vi "Dashboard Main - save.vi"() -> ()   [LabVIEW 2014]
uses:
  <vilib>/event_ctls.llb/eventvkey.ctl
  <vilib>/Utility/config.llb/NI_LVConfig.lvlib
  <vilib>/Utility/config.llb/Write Key (I32).vi
  <vilib>/Rock Robotics/WPI/Dashboard/WPI_DashboardLogging Global.vi
  <vilib>/Utility/config.llb/Write Key (String).vi
panel:
  in  "TCP":refnum<k5>
  in  "Rec Mode":enum32{"Stop", "Record", "Playback"}(radio)
  in  "Vision":u16(ring) items=["Camera Off", "USB Camera SW", "USB Camera HW", "IP Camera"]
  out "Camera IP":string
  out "Image Message":string="Timeout in Camera Communications"
  in  "Dashboard Tab":T1(tab)
  in  "Boolean":bool
  out "Low Battery":bool
  out "FMS":bool
  out "Teleop Mode":bool
  out "Auto Mode":bool
  out "Disabled":bool
  in  "Program":string
  in  "Camera Settings":T2={"Frame Rate"=30, "Compression"=30, "Size"=1} {"Frame Rate" scale=1.0..30.0; "Size" items=["640x480", "320x240", "160x120"]}
  out "Mode":T3(ring)=enum."Auto Disabled"
  in  "DB Camera Config":bool
  out "fps":dbl format="%#.1g"
  out "Mbps":dbl format="%#.1g"
  out "Mbps 2":bool
  in  "LCD Line 10":string caption="DB/String 0"
  in  "LCD Line 9":string caption="DB/String 0"
  in  "LCD Line 8":string caption="DB/String 0"
  in  "LCD Line 7":string caption="DB/String 0"
  in  "LCD Line 6":string caption="DB/String 0"
  in  "LCD Line 5":string caption="DB/String 0"
  in  "LCD Line 4":string caption="DB/String 0"
  in  "LCD Line 3":string caption="DB/String 0"
  in  "LCD Line 2":string caption="DB/String 0"
  in  "LCD Line 1":string caption="DB/String 0"
  in  "DB/String 9":string
  in  "DB/String 8":string
  in  "DB/String 7":string
  in  "DB/String 6":string
  in  "DB/String 5":string
  in  "DB/String 4":string
  in  "DB/String 3":string
  in  "DB/String 2":string
  in  "DB/String 1":string
  in  "DB/String 0":string
  in  "DB/Slider 0":dbl(slide) scale=0.0..5.0
  in  "DB/Slider 1":dbl(slide) scale=0.0..5.0
  in  "DB/Slider 2":dbl(slide) scale=0.0..5.0
  in  "DB/Slider 3":dbl(slide) scale=0.0..5.0
  out "DB/LED 3":bool
  out "DB/LED 2":bool
  out "DB/LED 1":bool
  out "DB/LED 0":bool
  in  "DB/Button 3":bool
  in  "DB/Button 2":bool
  in  "DB/Button 1":bool
  in  "DB/Button 0":bool caption="New Name"
  in  "Test Slider":dbl(slide) scale=0.0..100.0 scale format="%#_3g"
  in  "On/Off":bool caption="Solenoid"
  in  "Test Name":u16(ring) items=["Select the test to run...", "Example Test", "-------------------------------", "List of tests is built in robot code.", "Replace with your own automated tests."]
  in  "Test Tree":string(tree)
  in  "Motor":cluster{"Value":dbl, "Enable":bool} {"Value" scale=-1.0..1.0 scale format="%#_3g"}
  out "Progress":T4 {"Test Progress" scale=0.0..100.0}
  in  "Rev/Fwd":cluster{"Forward":bool, "Reverse":bool}
  in  "Test Ring":u16(ring) items=["Monochrome", "Color"]
  in  "Listbox":i32(listbox)
  out "Tree":string(tree)
  out "Camera Image":T5(plugin-control)
  # "Program:"
  # "Dashboard: 2015-02"
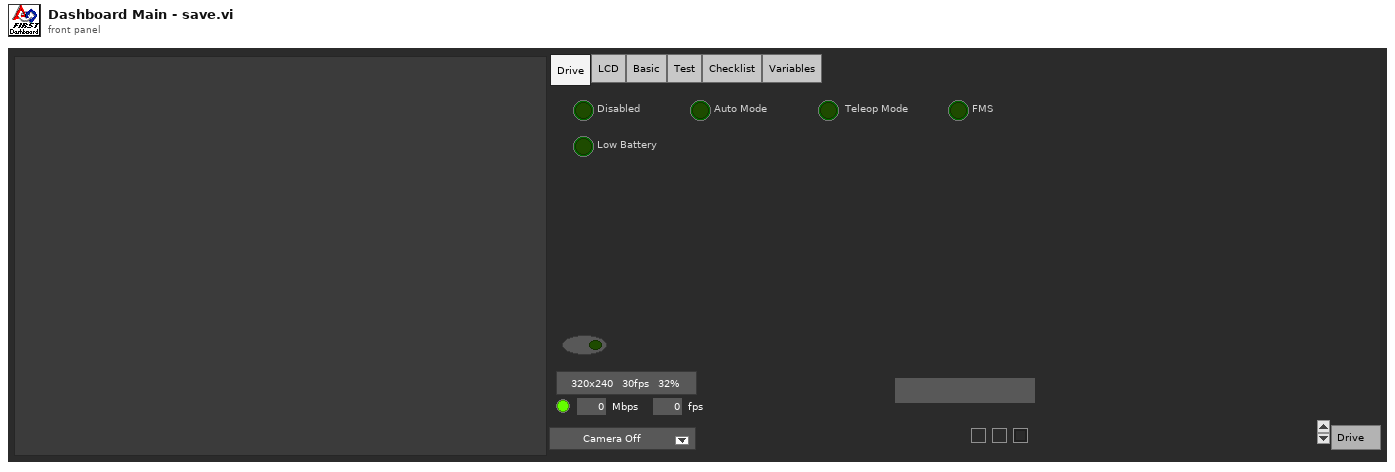
[diagram p1: front panel]
types:
  T1 = enum32{"Drive", "LCD", "Basic", "Test", "Checklist", "Variables"}
  T2 = cluster{"Frame Rate":i32, "Compression":i32, "Size":u16}
  T3 = enum8{"Tele-Op Disabled", "Tele-Op Enabled", "Auto Disabled", "Auto Enabled", "Test Disabled", "Test Enabled", "Disconnected", "No Code", "E-Stop"}
  T4 = cluster{"Test Progress":u8, "Test Progress Text":string}
  T5 = typedef "IMAQ Image.ctl" = refnum<image>
  T6 = enum32{"Drive", "Basic", "Custom", "Test", "Checklist", "Variables"}
  T7 = typedef "Image Type" = u32
  T8 = cluster{"Camera Image":refnum<vi>, "Dashboard Tab":refnum<vi>, "Vision":refnum<vi>, "Rec Mode":refnum<vi>, "Test Slider":refnum<vi>, "On/Off ":refnum<vi>, "Test Ring":refnum<vi>, "Rev/Fwd":refnum<vi>, "Test Name":refnum<vi>, "Motor":refnum<vi>, "Progress":refnum<vi>, "CheckList":refnum<vi>, "Tree":refnum<vi>, "Test Tree":refnum<vi>, void}
  T9 = cluster{"Error Strings":string, "Disable Counts":cluster{u16, u16}, "Rail Faults":cluster{u16, u16, u16}, "Robot IP":string, "DB Mode":u8, "Event Info":cluster{"Name":string, "Type":u8, "Number":u16, "Replay":u8}, "Camera Addr":string}
  T10 = cluster{"Storage":cluster{"Disk Free":u64, "RAM Block":u32, "RAM free":u32}, "CPU Utilization":cluster{"CPU % ISR":sgl, "CPU % Time Crit":sgl, "CPU % Timed Str":sgl, "CPU % High":sgl, "CPU % Above":sgl, "CPU % Normal":sgl, "CPU % Low":sgl}, "CAN":cluster{"% Bus Utilization":sgl, "Bus Off Cnt":u32, "TX_FIFO Full Cnt":u32, "Receive Error Cnt":u8, "Transmit Error Cnt":u8}, "HID":cluster{"HID Outputs":u32, "Rumble Low":u16, "Rumble High":u16}[]}
  T11 = cluster{"Status bits":cluster{"Test Mode":bool, "Autonomous":bool, "Enabled":bool, "Code Start":bool, "Brownout":bool, "Reserved 2":bool, "Reserved 3":bool, "E-Stop":bool}, "Code Trace":cluster{"Disabled":bool, "TeleOp":bool, "Auto":bool, "Test":bool}, "Controller Type":enum16{"unknown", "cRIO", "roboRio"}, "Code?":enum16{"unknown", "noCode", "code"}, "Battery V":dbl}
  T12 = cluster{"Control Bits":cluster{"TestMode":bool, "Autonomous":bool, "Enabled":bool, "FMS Present":bool, bool, bool, bool, "E-Stop":bool}, "Team Station ":u8, "Countdown":sgl, "Joystick Values":cluster{"Axes":dbl[], "Buttons":bool[], "POVs":i16[]}[]}
  T13 = cluster{"Axes":dbl[], "Buttons":bool[], "POVs":i16[]}[]
  T14 = cluster{"Axes":dbl[], "Buttons":bool[], "POVs":i16[]}
  T15 = typedef "NI_LVConfig.lvlib/Config Data RefNum.ctl" = refnum<k1>
  T16 = cluster{"Operation":enum16{"Update", "Clear"}, "Color Box":u32}[]
  T17 = typedef "eventvkey.ctl" = enum16{"ASCII", "Enter", "Return", "Shift", "Ctrl", "Alt", "Cmd", "Opt", "Caps", "NumLock", "Clear", "Break", "Up", "Down", "Left", "Right", "Insert", "Delete", "Home", "End", "PageUp", "PageDown", "Escape", "Help", "Pause", "ScrollLock", "F1", "F2", "F3", "F4", "F5", "F6", "F7", "F8", "F9", "F10", "F11", "F12", "F13", "F14", "F15", "F16", "F17", "F18", "F19", "F20", "F21", "F22", "F23", "F24", "Play", "VolumeUp", "VolumeDown", "Mute", "Two Byte Char"}
  T18 = cluster{"Image Size":bool, "Image Type":bool, "Pixel Value":bool, "ROI Information":bool, "Zoom Factor":bool}
  T19 = enum8{"Enabled", "Disabled", "Disabled and Grayed Out"}
  T20 = cluster{"Operation":enum16{"Update", "Clear"}, "Color Box":u32}
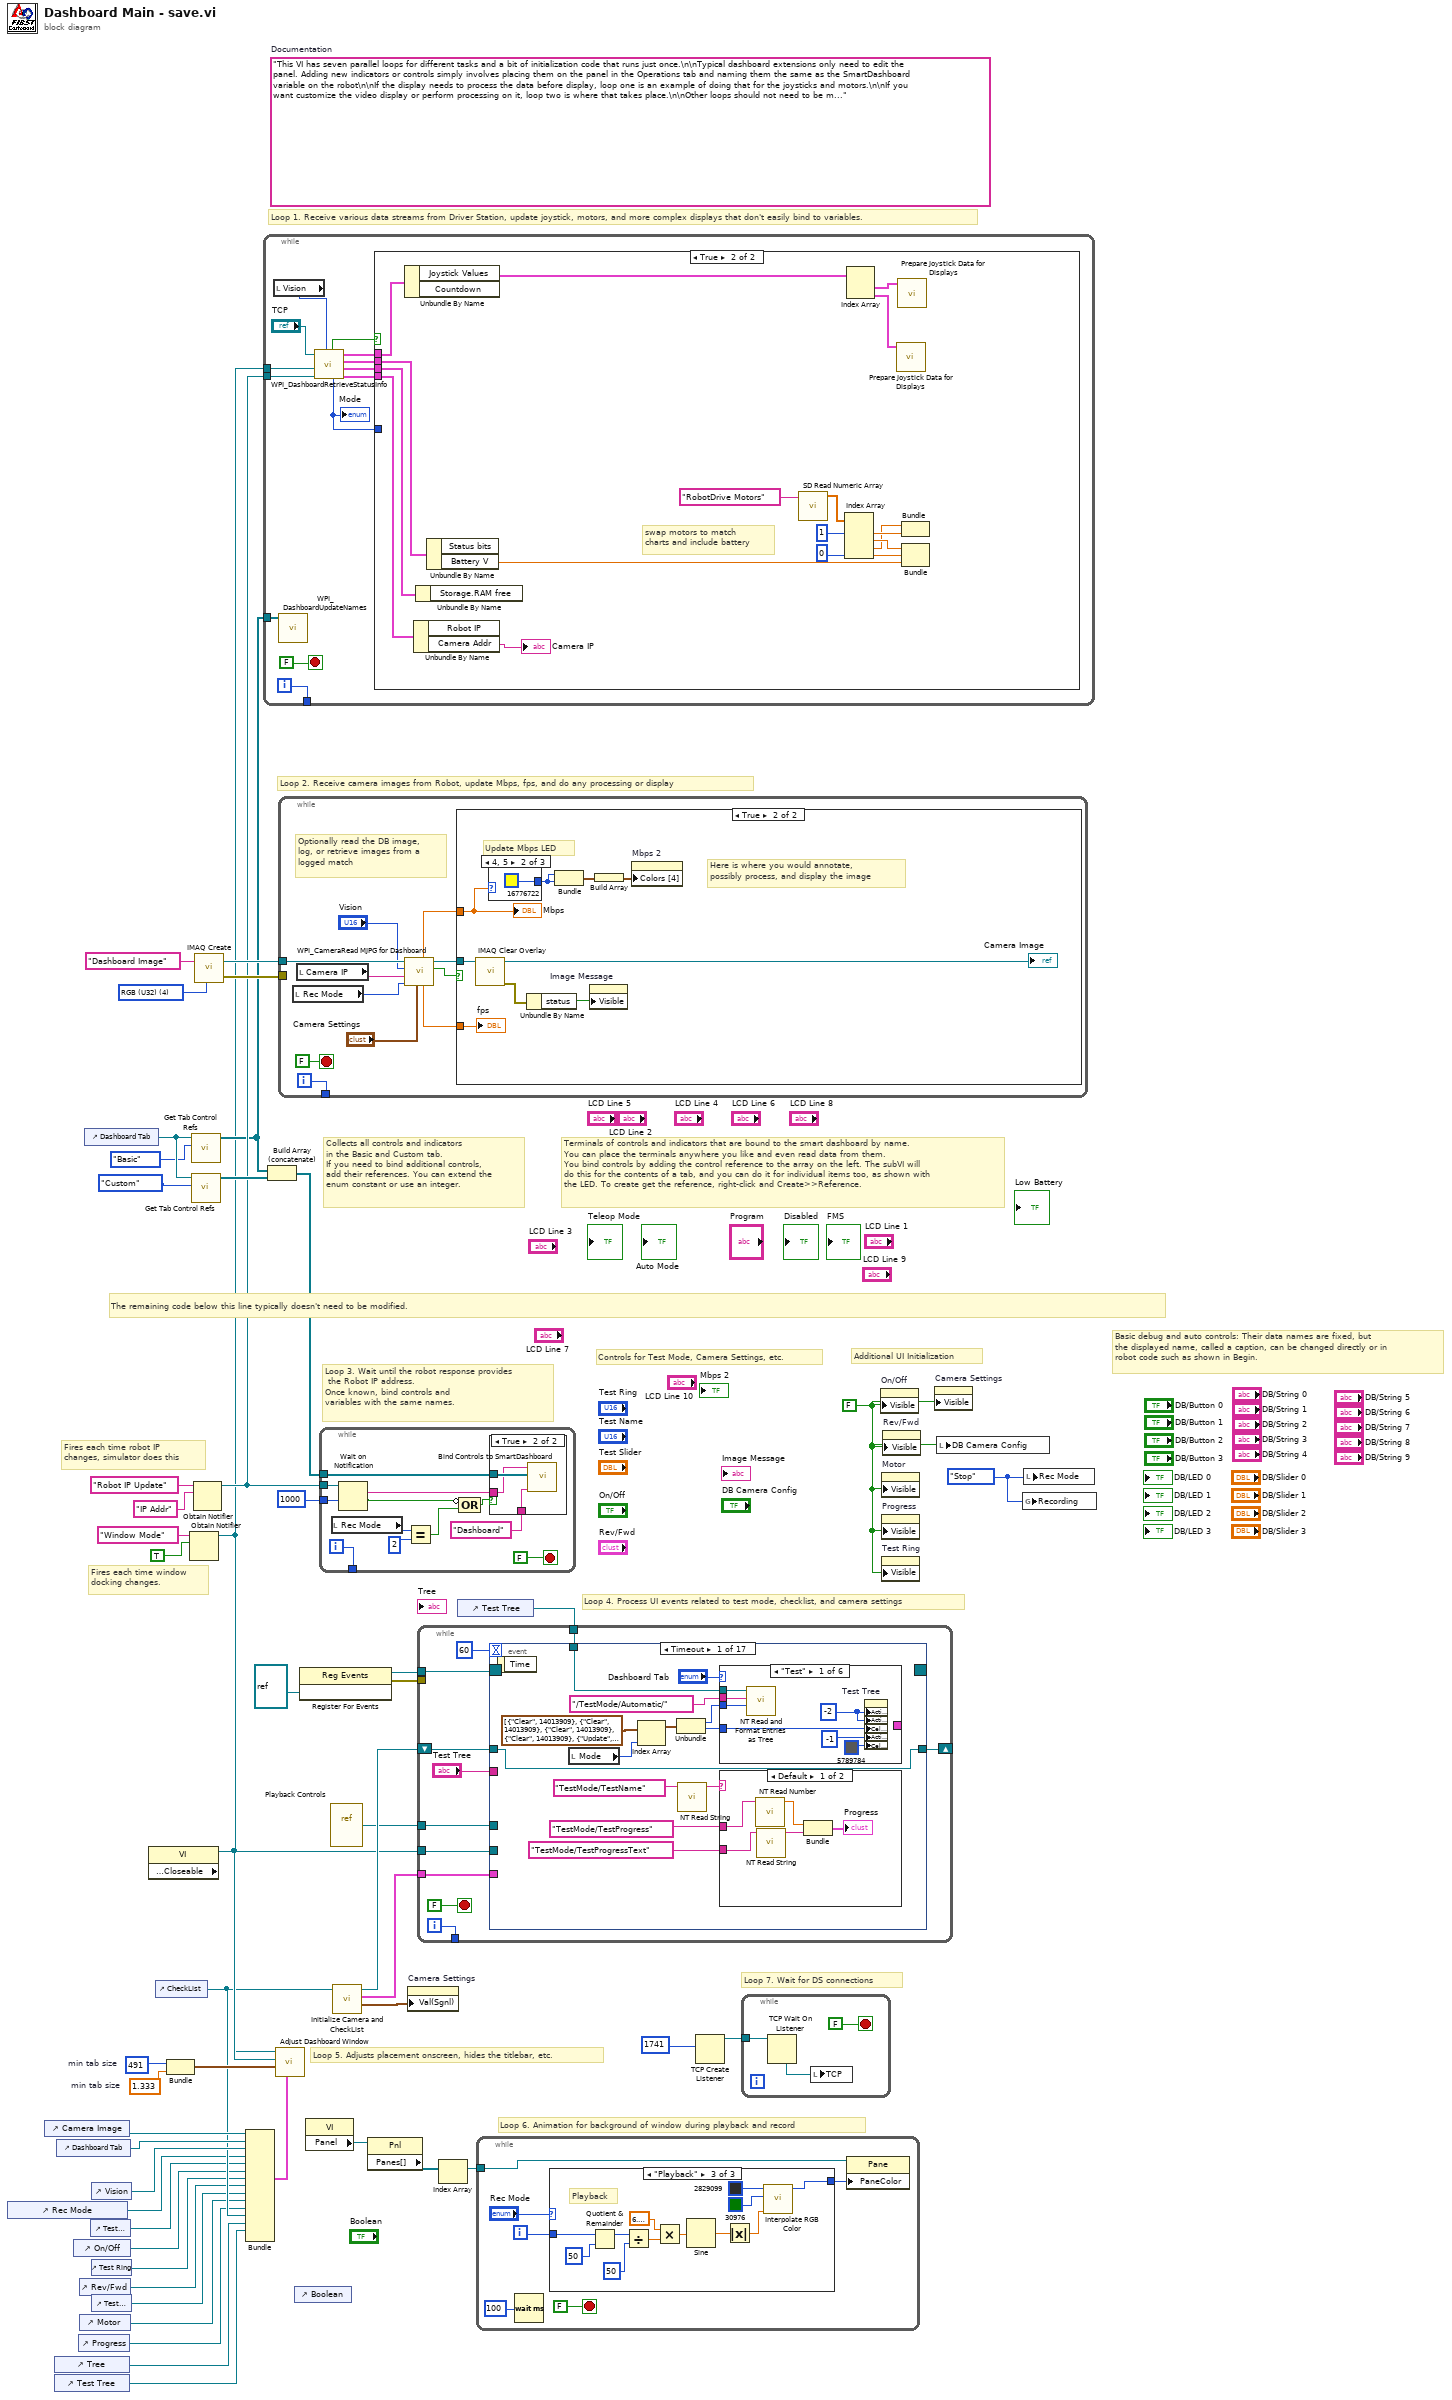
[diagram p0: block diagram]
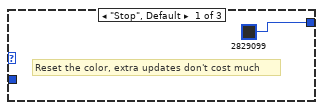
[diagram p3: hidden frame]
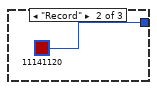
[diagram p4: hidden frame]
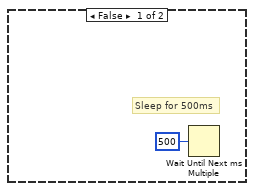
[diagram p6: hidden frame]
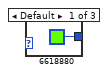
[diagram p7: hidden frame]
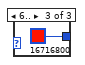
[diagram p8: hidden frame]
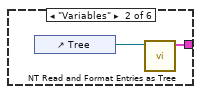
[diagram p9: hidden frame]
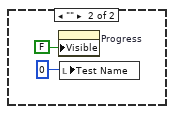
[diagram p14: hidden frame]
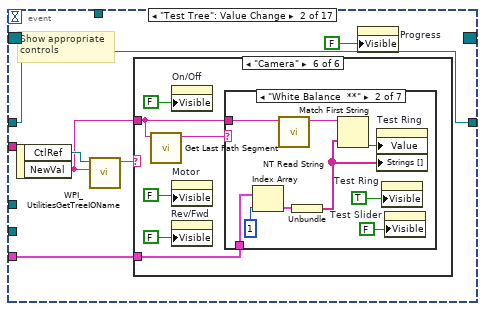
[diagram p15: hidden frame]
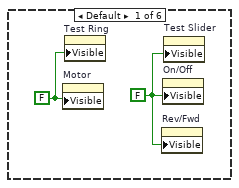
[diagram p16: hidden frame]
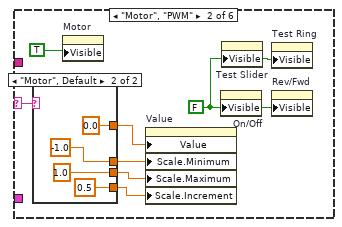
[diagram p17: hidden frame]
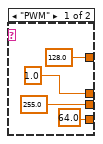
[diagram p18: hidden frame]
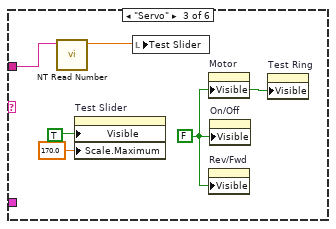
[diagram p19: hidden frame]
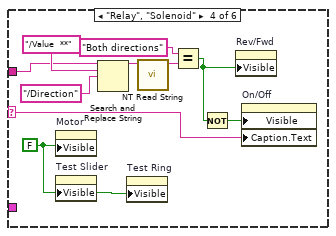
[diagram p20: hidden frame]
diagram:
  w23 = 491  # min tab size
  w22 = 1.333  # min tab size
  w31 = enum32{"Stop", "Record", "Playback"}."Stop" ("Rec Mode")
  w6 = FALSE ("Visible")
  (unwired) "This VI has seven parallel loops for different tasks and a bit of initialization code that runs just once.\n\nTypical dashboard extensions only need to edit the panel. Adding new indicators or controls simply involves placing them on the panel in the Operations tab and naming them the same as the SmartDashboard variable on the robot\n\nIf the display needs to process the data before display, loop one is an example of doing that for the joysticks and motors.\n\nIf you want customize the video display or perform processing on it, loop two is where that takes place.\n\nOther loops should not need to be modified. They are pretty standard, and document the task they perform."  # Documentation
  w51 = T7 4 items=["Grayscale (U8)", "Grayscale (I16)", "Grayscale (SGL)", "Complex (CSG)", "RGB (U32)", "HSL (U32)", "RGB (U64)"] ("Image Type")
  # "Loop 7. Wait for DS connections"
  # "Basic debug and auto controls: Their data names are fixed, but\nthe displayed name, called a caption, can be changed directly or in\nrobot code such as shown in Begin."
  # "Controls for Test Mode, Camera Settings, etc."
  # "Additional UI Initialization"
  # "Loop 6. Animation for background of window during playback and record"
  # "Fires each time robot IP\nchanges, simulator does this"
  # "Fires each time window\ndocking changes."
  # "Collects all controls and indicators\nin the Basic and Custom tab.\nIf you need to bind additional controls,\nadd their references. You can extend the\nenum constant or use an integer."
  # "The remaining code below this line typically doesn't need to be modified."
  # "Loop 4. Process UI events related to test mode, checklist, and camera settings"
  # "Terminals of controls and indicators that are bound to the smart dashboard by name.\nYou can place the terminals anywhere you like and even read data from them.\nYou bind controls by adding the control reference to the array on the left. The subVI will\ndo this for the contents of a tab, and you can do it for individual items too, as shown with\nthe LED. To create get the reference, right-click and Create>>Reference."
  # "Loop 3. Wait until the robot response provides\n the Robot IP address.\nOnce known, bind controls and\nvariables with the same names."
  # "Loop 5. Adjusts placement onscreen, hides the titlebar, etc."
  # "Loop 1. Receive various data streams from Driver Station, update joystick, motors, and more complex displays that don't easily bind to variables."
  # "Loop 2. Receive camera images from Robot, update Mbps, fps, and do any processing or display"
  n1 = control-ref of="Rec Mode"() -> (w12:refnum<vi>)
  n2 = control-ref of="Camera Image"() -> (w26:refnum<vi>)
  n3 = control-ref of="Tree"() -> (w16:refnum<vi>)
  n4 = control-ref of="Test Tree"() -> (w15:refnum<vi>)
  n5 = control-ref of="Dashboard Tab"() -> (w25:refnum<vi>)
  n6 = control-ref of="On/Off"() -> (w10:refnum<vi>)
  n7 = control-ref of="Progress"() -> (w7:refnum<vi>)
  n8 = control-ref of="Rev/Fwd"() -> (w8:refnum<vi>)
  n9 = control-ref of="Motor"() -> (w13:refnum<vi>)
  n10 = control-ref of="Dashboard Tab"() -> (w29:refnum<vi>)
  n11 = control-ref of="Test Slider"() -> (w11:refnum<vi>)
  n12 = control-ref of="Vision"() -> (w24:refnum<vi>)
  n13 = control-ref of="Test Ring"() -> (w9:refnum<vi>)
  n14 = control-ref of="Test Name"() -> (w14:refnum<vi>)
  n15 = property class="VI" props=["Front Panel.Closeable"]() -> (reference out=w30:refnum<vi>)  [unwired: 2 in, 2 out]
  n16 = control-ref of="CheckList"() -> (w17:refnum<vi>)
  n17 = Bundle("min tab size"=w23, "min tab size"=w22) -> (w21:cluster{"min tab size":i32, "min tab size":dbl})  [unwired: 1 in]
  n18 = Obtain Notifier(name (unnamed)="Window Mode", notification data type=TRUE) -> (notifier out=w3:refnum<notifier>)  [unwired: 2 in, 2 out]
  n19 = call <vilib>:"Get Tab Control Refs.vi"("Page Index"=T6."Basic" ("Dashboard Tab"), "TabControl in"=w29) -> ("ControlsOnPage"=w4:refnum<vi>[])  [unwired: 9 in]
  n20 = call <vilib>:"Get Tab Control Refs.vi"("Page Index"=T6."Custom" ("Dashboard Tab"), "TabControl in"=w29) -> ("ControlsOnPage"=w28:refnum<vi>[])  [unwired: 9 in]
  n21 = Obtain Notifier(name (unnamed)="Robot IP Update", notification data type="IP Addr" ("name (unnamed)")) -> (notifier out=w5:refnum<notifier>)  [unwired: 2 in, 2 out]
  n22 = call "IMAQ Create"("Image Name"="Dashboard Image", "Image Type"=w51) -> ("New Image"=w49:T5, "error out"=w48:errorcluster)  [unwired: 2 in, 1 out]
  n23 = Bundle("Camera Image"=w26, "Dashboard Tab"=w25, "Vision"=w24, "Rec Mode"=w12, "Test Slider"=w11, "On/Off"=w10, "Test Ring"=w9, "Rev/Fwd"=w8, "Test Name"=w14, "Motor"=w13, "Progress"=w7, "CheckList"=w17, "Tree"=w16, "Test Tree"=w15) -> (w18:T8)  [unwired: 2 in]
  n24 = while {
    tunnel: [w63] -> _
    tunnel: w5 -> [w57]
    tunnel: w4 -> [w56]
    tunnel: w3 -> [w52]
    i -> [w63]
    stop <- FALSE stop-if-true
    n25 = local read "Vision"() -> (w54:u16)
    n26 = call <vilib>:"WPI_DashboardUpdateNames.vi"("Controls on Tab"=w56) -> ()  [unwired: 11 in]
    n27 = call <vilib>:"WPI_DashboardRetrieveStatusInfo.vi"("Vision"=w54, "Binding Refnum"=w57, "Window Mode Notifier"=w52, "TCP Cnx"="TCP") -> ("Power and Errors"=w58:T9, "Robot Metrics"=w61:T10, "Status Info"=w62:T11, "Control Info"=w59:T12, "Robot Mode"=w55:T3, "Process?"=w60:bool)  [unwired: 2 in]
    "Mode" <- w55
    n28 = case shown="True" w60 {
      tunnel: w62 -> [_ w81]
      tunnel: w61 -> [_ w80]
      tunnel: w59 -> [_ w79]
      tunnel: w58 -> [_ w78]
      tunnel: w55 -> [_ _]
      frame False {
      }
      frame True {
        # "swap motors to match\ncharts and include battery"
        n29 = Unbundle By Name(w79) -> ("Joystick Values"=w68:T13)  [unwired: 1 out]
        n30 = Unbundle By Name(w78) -> ("Camera Addr"=→"Camera IP":string)  [unwired: 1 out]
        n31 = Unbundle By Name(w80) -> ()  [unwired: 1 out]
        n32 = Unbundle By Name(w81) -> ("Battery V"=w69:dbl)  [unwired: 1 out]
        n33 = call <vilib>:"SD Read Numeric Array.vi"("Name"="RobotDrive Motors") -> ("Numeric Array"=w71:dbl[])  [unwired: 8 in, 2 out]
        n34 = Index Array(array=w71, index #1=1, index #4=0) -> (element #1=w73:dbl, element #2=w74:dbl, element #3=w72:dbl, element #4=w77:dbl)  [unwired: 2 in]
        n35 = Index Array(array=w68) -> (element #1=w67:T14, element #2=w65:T14)  [unwired: 2 in]
        n36 = call "Prepare Joystick Data for Displays.vi"("Joystick Values"=w65) -> ()  [unwired: 8 in, 3 out]
        n37 = call "Prepare Joystick Data for Displays.vi"("Joystick Values"=w67) -> ()  [unwired: 8 in, 3 out]
        n38 = Bundle("Numeric"=w72, "Numeric"=w73) -> ()  [unwired: 1 in, 1 out]
        n39 = Bundle("Numeric"=w74, "Numeric"=w77, "Battery V"=w69) -> ()  [unwired: 1 in, 1 out]
      }
    }
  }
  n40 = Build Array (concatenate)(w4, w28) -> (w27:refnum<vi>[])
  n41 = call "Adjust Dashboard Window.vi"("Sizing Refnums"=w18, "Size Constraints"=w21, "VI"=w30, "Notifier in"=w3) -> ()  [unwired: 8 in]
  n42 = while {
    tunnel: w49 -> [w90]
    tunnel: w48 -> [_]
    tunnel: [w91] -> _
    i -> [w91]
    stop <- FALSE stop-if-true
    # "Optionally read the DB image,\nlog, or retrieve images from a\nlogged match"
    n43 = local read "Rec Mode"() -> (w84:enum32{"Stop", "Record", "Playback"})
    n44 = local read "Camera IP"() -> (w82:string)
    n45 = call <vilib>:"WPI_CameraRead MJPG for Dashboard.vi"("Camera Settings"="Camera Settings", "Rec Mode"=w84, "Camera IP"=w82, "Camera Mode"="Vision", "Refnum in"=w90) -> ("Active"=w88:bool, "Refnum out"=w89:T5, "FPS"=w87:dbl, "Bandwidth (Mbps)"=w86:dbl)  [unwired: 3 in]
    n46 = case shown="True" w88 {
      tunnel: w89 -> [_ w97]
      tunnel: w86 -> [_ w96]
      tunnel: w87 -> [_ w94]
      frame False {
        # "Sleep for 500ms"
        n47 = Wait Until Next ms Multiple(millisecond multiple=u32 500) -> ()  [unwired: 1 out]
      }
      frame True {
        # "Here is where you would annotate,\npossibly process, and display the image"
        # "Update Mbps LED"
        n48 = call "IMAQ Clear Overlay"("Image"=w97) -> ("error out"=w101:errorcluster, "Image Out"=→"Camera Image":T5)  [unwired: 2 in, 7 out]
        n49 = case shown="4, 5" w96 {
          tunnel: [u32 6618880 ("Color Box") u32 16776722 ("Color Box") u32 16716800 ("Color Box")] -> w98
          frame Default {
          }
          frame 4, 5 {
          }
          frame 6.. {
          }
        }
        n50 = Unbundle By Name(w101) -> ("status"=w102:bool)
        n51 = Bundle("Color Box"=w98, "Color Box"=w98) -> (w100:cluster{"Color Box":u32, "Color Box":u32})  [unwired: 1 out]
        n52 = property on="Image Message" class="Str"("Visible"=w102) -> ()  [unwired: 2 in, 2 out]
        n53 = Build Array(w100) -> (w99:cluster{"Color Box":u32, "Color Box":u32}[])
        n54 = property on="Mbps 2" class="Bool (strict)"("Colors [4]"=w99) -> ()  [unwired: 2 in, 2 out]
        "Mbps" <- w96
        "fps" <- w94
      }
    }
  }
  n55 = control-ref of="Boolean"() -> ()  [unwired: 1 out]
  n56 = register-events(refnum<vi> refnum) -> (reference out=w35:refnum<event-registration>, error out=w34:errorcluster)  [unwired: 2 in]
  n57 = property class="VI"() -> ("Panel"=w38:refnum<vi>)  [unwired: 2 in, 2 out]
  n58 = while {
    tunnel: w27 -> [w117]
    tunnel: w5 -> [w115]
    tunnel: [w113] -> _
    tunnel: u32 1000 ("milliseconds to wait") -> [w112]
    i -> [w113]
    stop <- FALSE stop-if-true
    n59 = local read "Rec Mode"() -> (w108:enum32{"Stop", "Record", "Playback"})
    n60 = Wait on Notification(notifier=w115, timeout in ms (-1)=w112) -> (notification=w114:string, timed out?=w110:bool)  [unwired: 2 in, 2 out]
    n61 = Equal?(x=w108, y=u16 2 ("Rec Mode")) -> (x = y?=w109:bool)
    n62 = Compound Arithmetic op=OR(invert w110, w109) -> (w111:bool)
    n63 = case shown="True" w111 {
      tunnel: w117 -> [_ w120]
      tunnel: w114 -> [_ w119]
      tunnel: "Dashboard" -> [_ w118]
      frame False {
      }
      frame True {
        n64 = call <vilib>:"Bind Controls to SmartDashboard.vi"("Client Name"=w118, "Bound Control Refs"=w120, "Server IP Address"=w119) -> ()  [unwired: 9 in]
      }
    }
  }
  n65 = vi-ref "Playback Controls.vi"() -> (w36:refnum<vi>)
  n66 = call "Initialize Camera and CheckList.vi"("ListBox in"=w17) -> ("Cluster"=w42:cluster{"value":i32, "value":i32, "index":i32}, "Array"=w43:cluster{string[]}[], "File Refnum"=w41:T15)  [unwired: 8 in]
  n67 = property class="Pnl"(reference=w38) -> ("Panes[]"=w39:refnum<vi>[])  [unwired: 1 in, 2 out]
  n68 = property on="Camera Settings" class="Clust (strict)"("Val(Sgnl)"=w42) -> ()  [unwired: 2 in, 2 out]
  n69 = Index Array(array=w39) -> (element=w37:refnum<vi>)  [unwired: 1 in]
  n70 = control-ref of="Test Tree"() -> (w40:refnum<vi>)
  n71 = while {
    tunnel: w43 -> [w128]
    shift-right: [w127] -> _
    shift-left: w41 -> [w126]
    tunnel: [w125] -> _
    tunnel: w40 -> [w124]
    tunnel: w36 -> [w123]
    tunnel: w35 -> [w122]
    tunnel: w34 -> [_]
    tunnel: w30 -> [w121]
    i -> [w125]
    stop <- FALSE stop-if-true
    n72 = event shown="[0] Timeout" {
      selector: w122 -> [_ _ _ _ _ _ _ _ _ _ _ _ _ _ _ _ _]
      dyn-events: [_ _ _ _ _ _ _ _ _ _ _ _ _ w366 _ _ _] -> _
      timeout: u32 60 ("milliseconds to wait") -> [_ _ _ _ _ _ _ _ _ _ _ _ _ _ _ _ _]
      tunnel: w124 -> [w140 _ _ _ _ _ _ _ _ _ _ _ _ _ _ _ _]
      tunnel: "Test Tree" -> [_ _ _ _ _ _ _ _ w335 w343 w345 w349 w357 _ _ _ _]
      tunnel: w128 -> [_ w162 _ _ _ _ w299 w329 _ _ _ _ _ _ _ _ _]
      tunnel: [w136 w161 w260 w265 w273 w285 w298 w322 w334 w341 w344 w348 w356 w368 w382 w383 w393] -> w127
      tunnel: w126 -> [w136 w161 w260 w265 w273 w285 w297 w322 w334 w341 w344 w348 w356 w368 w382 w383 w393]
      tunnel: w123 -> [_ _ _ _ _ _ _ _ _ _ _ _ _ w369 _ w386 _]
      tunnel: w121 -> [_ _ _ _ _ _ _ _ _ _ _ _ _ w364 _ _ _]
      event Timeout {
        n73 = event-data() -> ()  [unwired: 1 in, 1 out]
        n74 = local read "Mode"() -> (w139:T3)
        n75 = Index Array(array=T16 [{"Operation"=enum."Clear", "Color Box"=14013909}, {"Operation"=enum."Clear", "Color Box"=14013909}, {"Operation"=enum."Clear", "Color Box"=14013909}, {"Operation"=enum."Clear", "Color Box"=14013909}, {"Operation"=enum."Update", "Color Box"=14013909}, {"Operation"=enum."Update", "Color Box"=16777215}, {"Operation"=enum."Clear", "Color Box"=14013909}, {"Operation"=enum."Clear", "Color Box"=14013909}, {"Operation"=enum."Clear", "Color Box"=14013909}], index=w139) -> (element=w134:T20)
        n76 = Unbundle(w134) -> ("Operation"=w133:enum16{"Update", "Clear"}, "Color Box"=w132:u32)
        n77 = call <vilib>:"NT Read String.vi"("Name"="TestMode/TestName") -> ("String"=w143:string)  [unwired: 9 in, 1 out]
        n78 = case shown="\"Test\"" "Dashboard Tab" {
          tunnel: w140 -> [w151 _ _ _ _ _]
          tunnel: "/TestMode/Automatic/" ("Name Pattern") -> [w150 _ _ _ _ _]
          tunnel: w133 -> [w149 _ _ _ _ _]
          tunnel: [_ w153 _ _ _ _] -> _
          tunnel: w132 -> [w145 _ _ _ _ _]
          frame "Test" {
            w148 = -2 ("Active Item:Row Number")
            n79 = call <vilib>:"NT Read and Format Entries as Tree.vi"("Operation"=w149, "Name Pattern"=w150, "Tree Refnum"=w151) -> ()  [unwired: 7 in, 2 out]
            n80 = property on="Test Tree" class="Tree (strict)"("Active Item Row Number"=w148, "ActiveColNum"=w148, "CellBG"=w145, "Active Item Row Number"=-1 ("Active Item:Row Number"), "CellBG"=u32 5789784 ("Color Box")) -> ()  [unwired: 2 in, 2 out]
          }
          frame "Variables" {
            n81 = control-ref of="Tree"() -> (w152:refnum<vi>)
            n82 = call <vilib>:"NT Read and Format Entries as Tree.vi"("Tree Refnum"=w152) -> ("Formatted Strings"=w153:cluster{"Name":string, "Value":string}[])  [unwired: 9 in, 1 out]
          }
          frame "Checklist" {
          }
          frame "Basic" {
          }
          frame "LCD" {
          }
          frame "Drive" {
          }
        }
        n83 = case shown="Default" w143 {
          tunnel: "TestMode/TestProgress" ("Name") -> [w155 _]
          tunnel: "TestMode/TestProgressText" ("Name") -> [w154 _]
          frame Default {
            n84 = call <vilib>:"NT Read Number.vi"("Name"=w155) -> ("Numeric"=w156:dbl)  [unwired: 9 in, 1 out]
            n85 = call <vilib>:"NT Read String.vi"("Name"=w154) -> ("String"=w157:string)  [unwired: 9 in, 1 out]
            n86 = Bundle("Numeric"=w156, "String"=w157) -> (→"Progress":cluster{"Numeric":dbl, "String":string})  [unwired: 1 in]
          }
          frame "" {
            n87 = property on="Progress" class="Clust (strict)"("Visible"=FALSE) -> ()  [unwired: 2 in, 2 out]
            n88 = local write "Test Name"(u16 0) -> ()
          }
        }
      }
      event "Test Tree": Value Change {
        # "Show appropriate\ncontrols"
        n89 = event-data() -> ("CtlRef"=w165:refnum<vi>, "NewVal"=w163:string)  [unwired: 1 in]
        n90 = call <vilib>:"WPI_UtilitiesGetTreeIOName.vi"("NewVal"=w163, "TreeControl in"=w165) -> ("I/O Name"=w166:string)  [unwired: 9 in]
        n91 = case shown="\"Camera\"" w166 {
          selector: w166 -> [_ w173 _ w191 w200 _]
          tunnel: w163 -> [_ _ w188 w190 _ w207]
          tunnel: w162 -> [_ _ _ _ _ w206]
          frame Default {
            w168 = FALSE ("Visible")
            w167 = FALSE ("Visible")
            n92 = property on="Motor" class="Clust (strict)"("Visible"=w167) -> ()  [unwired: 2 in, 2 out]
            n93 = property on="Test Ring" class="Ring (strict)"("Visible"=w167) -> ()  [unwired: 2 in, 2 out]
            n94 = property on="Rev/Fwd" class="Clust (strict)"("Visible"=w168) -> ()  [unwired: 2 in, 2 out]
            n95 = property on="On/Off" class="Bool (strict)"("Visible"=w168) -> ()  [unwired: 2 in, 2 out]
            n96 = property on="Test Slider" class="Slide (strict)"("Visible"=w168) -> ()  [unwired: 2 in, 2 out]
          }
          frame "Motor", "PWM" {
            w174 = FALSE ("Visible")
            n97 = case shown="\"Motor\", Default" w173 {
              tunnel: [1.0 ("Value") -1.0 ("Value")] -> w172
              tunnel: [255.0 ("Value") 1.0 ("Value")] -> w171
              tunnel: [128.0 ("Value") 0.0 ("Value")] -> w170
              tunnel: [64.0 ("Value") 0.5 ("Value")] -> w169
              frame "PWM" {
              }
              frame "Motor", Default {
              }
            }
            n98 = property on="Motor" class="Clust (strict)"("Visible"=TRUE) -> ()  [unwired: 2 in, 2 out]
            n99 = property on="Value" class="Slide (strict)"("Value"=w170, "Scale.Minimum"=w172, "Scale.Maximum"=w171, "Scale.Increment"=w169) -> ()  [unwired: 2 in, 2 out]
            n100 = property on="On/Off" class="Bool (strict)"("Visible"=w174) -> ()  [unwired: 2 in, 2 out]
            n101 = property on="Test Slider" class="Slide (strict)"("Visible"=w174) -> ()  [unwired: 2 in, 2 out]
            n102 = property on="Test Ring" class="Ring (strict)"("Visible"=w174) -> ()  [unwired: 2 in, 2 out]
            n103 = property on="Rev/Fwd" class="Clust (strict)"("Visible"=w174) -> ()  [unwired: 2 in, 2 out]
          }
          frame "Servo" {
            w186 = FALSE ("Visible")
            n104 = call <vilib>:"NT Read Number.vi"("Name"=w188) -> ("Numeric"=w187:dbl)  [unwired: 9 in, 1 out]
            n105 = property on="Test Slider" class="Slide (strict)"("Visible"=TRUE, "Scale.Maximum"=170.0 ("Scale.Range:Maximum")) -> ()  [unwired: 2 in, 2 out]
            n106 = local write "Test Slider"(w187) -> ()
            n107 = property on="Motor" class="Clust (strict)"("Visible"=w186) -> ()  [unwired: 2 in, 2 out]
            n108 = property on="Rev/Fwd" class="Clust (strict)"("Visible"=w186) -> ()  [unwired: 2 in, 2 out]
            n109 = property on="On/Off" class="Bool (strict)"("Visible"=w186) -> ()  [unwired: 2 in, 2 out]
            n110 = property on="Test Ring" class="Ring (strict)"("Visible"=w186) -> ()  [unwired: 2 in, 2 out]
          }
          frame "Relay", "Solenoid" {
            w189 = FALSE ("Visible")
            n111 = property on="Motor" class="Clust (strict)"("Visible"=w189) -> ()  [unwired: 2 in, 2 out]
            n112 = property on="Test Slider" class="Slide (strict)"("Visible"=w189) -> ()  [unwired: 2 in, 2 out]
            n113 = Search and Replace String(input string=w190, search string="/Value  **", replace string="/Direction") -> (result string=w196:string)  [unwired: 5 in, 3 out]
            n114 = property on="Test Ring" class="Ring (strict)"("Visible"=w189) -> ()  [unwired: 2 in, 2 out]
            n115 = call <vilib>:"NT Read String.vi"("Name"=w196) -> ("String"=w194:string)  [unwired: 9 in, 1 out]
            n116 = Equal?(x="Both directions", y=w194) -> (x = y?=w192:bool)
            n117 = Not(x=w192) -> (.not. x?=w193:bool)
            n118 = property on="Rev/Fwd" class="Clust (strict)"("Visible"=w192) -> ()  [unwired: 2 in, 2 out]
            n119 = property on="On/Off" class="Bool (strict)"("Visible"=w193, "Caption.Text"=w191) -> ()  [unwired: 2 in, 2 out]
          }
          frame "Compressor", "Digital Out" {
            w199 = FALSE ("Visible")
            # "Get direction and finish"
            n120 = property on="Motor" class="Clust (strict)"("Visible"=w199) -> ()  [unwired: 2 in, 2 out]
            n121 = property on="Test Slider" class="Slide (strict)"("Visible"=w199) -> ()  [unwired: 2 in, 2 out]
            n122 = property on="Test Ring" class="Ring (strict)"("Visible"=w199) -> ()  [unwired: 2 in, 2 out]
            n123 = property on="On/Off" class="Bool (strict)"("Visible"=TRUE, "Caption.Text"=w200) -> ()  [unwired: 2 in, 2 out]
            n124 = property on="Rev/Fwd" class="Clust (strict)"("Visible"=FALSE) -> ()  [unwired: 2 in, 2 out]
          }
          frame "Camera" {
            n125 = call <vilib>:"Get Last Path Segment.vi"("String in"=w207) -> ("String out"=w208:string)  [unwired: 10 in]
            n126 = property on="On/Off" class="Bool (strict)"("Visible"=FALSE) -> ()  [unwired: 2 in, 2 out]
            n127 = property on="Motor" class="Clust (strict)"("Visible"=FALSE) -> ()  [unwired: 2 in, 2 out]
            n128 = property on="Rev/Fwd" class="Clust (strict)"("Visible"=FALSE) -> ()  [unwired: 2 in, 2 out]
            n129 = case shown="\"White Balance  **\"" w208 {
              tunnel: w207 -> [w214 w223 w232 w241 w250 _ w256]
              tunnel: w206 -> [w212 w220 w229 w238 w247 _ _]
              frame "Size  **" {
                n130 = Index Array(array=w212) -> (element=w211:cluster{string[]})  [unwired: 1 in]
                n131 = call <vilib>:"NT Read String.vi"("Name"=w214) -> ("String"=w213:string)  [unwired: 9 in, 1 out]
                n132 = Unbundle(w211) -> (w209:string[])
                n133 = Match First String(2:w209, 3:w213) -> (0:w210:i32)  [unwired: 1 out]
                n134 = property on="Test Ring" class="Ring (strict)"("Value"=w210, "Strings []"=w209) -> ()  [unwired: 2 in, 2 out]
                n135 = property on="Test Ring" class="Ring (strict)"("Visible"=TRUE) -> ()  [unwired: 2 in, 2 out]
                n136 = property on="Test Slider" class="Slide (strict)"("Visible"=FALSE) -> ()  [unwired: 2 in, 2 out]
              }
              frame "White Balance  **" {
                n137 = Index Array(array=w220, index=1) -> (element=w221:cluster{string[]})
                n138 = call <vilib>:"NT Read String.vi"("Name"=w223) -> ("String"=w222:string)  [unwired: 9 in, 1 out]
                n139 = Unbundle(w221) -> (w218:string[])
                n140 = Match First String(2:w218, 3:w222) -> (0:w217:i32)  [unwired: 1 out]
                n141 = property on="Test Ring" class="Ring (strict)"("Value"=w217, "Strings []"=w218) -> ()  [unwired: 2 in, 2 out]
                n142 = property on="Test Ring" class="Ring (strict)"("Visible"=TRUE) -> ()  [unwired: 2 in, 2 out]
                n143 = property on="Test Slider" class="Slide (strict)"("Visible"=FALSE) -> ()  [unwired: 2 in, 2 out]
              }
              frame "Exposure  **" {
                n144 = Index Array(array=w229, index=2) -> (element=w230:cluster{string[]})
                n145 = call <vilib>:"NT Read String.vi"("Name"=w232) -> ("String"=w231:string)  [unwired: 9 in, 1 out]
                n146 = Unbundle(w230) -> (w226:string[])
                n147 = Match First String(2:w226, 3:w231) -> (0:w227:i32)  [unwired: 1 out]
                n148 = property on="Test Ring" class="Ring (strict)"("Value"=w227, "Strings []"=w226) -> ()  [unwired: 2 in, 2 out]
                n149 = property on="Test Ring" class="Ring (strict)"("Visible"=TRUE) -> ()  [unwired: 2 in, 2 out]
                n150 = property on="Test Slider" class="Slide (strict)"("Visible"=FALSE) -> ()  [unwired: 2 in, 2 out]
              }
              frame "Exposure Priority  **" {
                n151 = Index Array(array=w238, index=3) -> (element=w239:cluster{string[]})
                n152 = call <vilib>:"NT Read String.vi"("Name"=w241) -> ("String"=w240:string)  [unwired: 9 in, 1 out]
                n153 = Unbundle(w239) -> (w235:string[])
                n154 = Match First String(2:w235, 3:w240) -> (0:w236:i32)  [unwired: 1 out]
                n155 = property on="Test Ring" class="Ring (strict)"("Value"=w236, "Strings []"=w235) -> ()  [unwired: 2 in, 2 out]
                n156 = property on="Test Ring" class="Ring (strict)"("Visible"=TRUE) -> ()  [unwired: 2 in, 2 out]
                n157 = property on="Test Slider" class="Slide (strict)"("Visible"=FALSE) -> ()  [unwired: 2 in, 2 out]
              }
              frame "Color Enable  **" {
                n158 = Index Array(array=w247, index=4) -> (element=w248:cluster{string[]})
                n159 = call <vilib>:"NT Read String.vi"("Name"=w250) -> ("String"=w249:string)  [unwired: 9 in, 1 out]
                n160 = Unbundle(w248) -> (w244:string[])
                n161 = Match First String(2:w244, 3:w249) -> (0:w245:i32)  [unwired: 1 out]
                n162 = property on="Test Ring" class="Ring (strict)"("Value"=w245, "Strings []"=w244) -> ()  [unwired: 2 in, 2 out]
                n163 = property on="Test Ring" class="Ring (strict)"("Visible"=TRUE) -> ()  [unwired: 2 in, 2 out]
                n164 = property on="Test Slider" class="Slide (strict)"("Visible"=FALSE) -> ()  [unwired: 2 in, 2 out]
              }
              frame Default {
                n165 = property on="Test Ring" class="Ring (strict)"("Visible"=FALSE) -> ()  [unwired: 2 in, 2 out]
                n166 = property on="Test Slider" class="Slide (strict)"("Visible"=FALSE) -> ()  [unwired: 2 in, 2 out]
              }
              frame "Brightness  **", "Color Level  **", "Compression  **", "FPS  **", "Sharpness  **" {
                n167 = call <vilib>:"NT Read Number.vi"("Name"=w256) -> ("Numeric"=w255:dbl)  [unwired: 9 in, 1 out]
                n168 = local write "Test Slider"(w255) -> ()
                n169 = property on="Test Slider" class="Slide (strict)"("Visible"=TRUE, "Scale.Maximum"=100.0 ("Scale.Range:Maximum")) -> ()  [unwired: 2 in, 2 out]
                n170 = property on="Test Ring" class="Ring (strict)"("Visible"=FALSE) -> ()  [unwired: 2 in, 2 out]
              }
            }
          }
        }
        n171 = property on="Progress" class="Clust (strict)"("Visible"=FALSE) -> ()  [unwired: 2 in, 2 out]
      }
      event "Test Name": Mouse Enter {
        # "Populate the ring with the list of tests"
        n172 = event-data() -> ()  [unwired: 1 in, 1 out]
        n173 = call <vilib>:"NT Read String Array.vi"("Name"="TestMode/TestList") -> ("String Array"=w264:string[])  [unwired: 9 in, 1 out]
        n174 = Build Array (concatenate)("Select the test to run...", w264) -> (w263:string[])
        n175 = property on="Test Name" class="Ring (strict)"("Strings []"=w263) -> ()  [unwired: 2 in, 2 out]
      }
      event "Test Name": Value Change {
        w266 = FALSE ("Visible")
        # "Tell the robot the test name to run"
        n176 = event-data() -> ("NewVal"=w270:u16)  [unwired: 1 in]
        n177 = property on="Test Name" class="Ring (strict)"() -> ("Strings []"=w271:string[])  [unwired: 2 in, 2 out]
        n178 = local write "Progress"(T4 {"Test Progress"=0, "Test Progress Text"=""} ("Progress")) -> ()
        n179 = Index Array(array=w271, index=w270) -> (element=w269:string)
        n180 = call <vilib>:"NT Write String.vi"("String"=w269, "Name"="TestMode/TestName") -> ()  [unwired: 9 in, 1 out]
        n181 = property on="Progress" class="Clust (strict)"("Visible"=TRUE) -> ()  [unwired: 2 in, 2 out]
        n182 = property on="Motor" class="Clust (strict)"("Visible"=w266) -> ()  [unwired: 2 in, 2 out]
        n183 = property on="Test Slider" class="Slide (strict)"("Visible"=w266) -> ()  [unwired: 2 in, 2 out]
        n184 = property on="On/Off" class="Bool (strict)"("Visible"=w266) -> ()  [unwired: 2 in, 2 out]
        n185 = property on="Rev/Fwd" class="Clust (strict)"("Visible"=w266) -> ()  [unwired: 2 in, 2 out]
        n186 = property on="Test Ring" class="Ring (strict)"("Visible"=w266) -> ()  [unwired: 2 in, 2 out]
      }
      event "Listbox": Double Click {
        # "Shift clears all"
        # "Update symbols on the listbox"
        n187 = event-data() -> ("PlatMods.Shift"=w274:bool, "Row"=w276:i32)  [unwired: 1 in]
        n188 = case shown="True" w274 {
          tunnel: w276 -> [w280 _]
          tunnel: 1 -> [w279 _]
          frame False {
            n189 = property on="Listbox" class="LstBox (strict)"() -> ("Item Symbols"=w278:i32[])  [unwired: 2 in, 2 out]
            n190 = Replace Array Subset(array=w278, new element=w279, index=w280) -> (w277:i32[])
            n191 = property on="Listbox" class="LstBox (strict)"("Item Symbols"=w277) -> ()  [unwired: 2 in, 2 out]
          }
          frame True {
            w281 = 0 ("Top Row")
            n192 = property on="Listbox" class="LstBox (strict)"() -> ("Number of Rows"=w283:u32)  [unwired: 2 in, 2 out]
            n193 = Initialize Array(0, w283) -> (w282:i32[])
            n194 = property on="Listbox" class="LstBox (strict)"("Top Row"=w281, "Value"=w281, "Item Symbols"=w282) -> ()  [unwired: 2 in, 2 out]
          }
        }
      }
      event "Listbox": Key Down {
        # "Update symbols on the listbox\nLeft and right keys check and uncheck"
        n195 = event-data() -> ("VKey"=w287:T17)  [unwired: 1 in]
        n196 = case shown="\"Left\", \"Right\"" w287 {
          selector: w287 -> [w292 _]
          tunnel: eventvkey."Left" ("VKey") -> [w290 _]
          frame "Left", "Right" {
            n197 = Equal?(x=w290, y=w292) -> (x = y?=w291:bool)
            n198 = Select(t=0, s=w291, f=1) -> (s? t:f=w293:i32)
            n199 = property on="Listbox" class="LstBox (strict)"() -> ("Item Symbols"=w296:i32[])  [unwired: 2 in, 2 out]
            n200 = Replace Array Subset(array=w296, new element=w293, index="Listbox") -> (w295:i32[])
            n201 = property on="Listbox" class="LstBox (strict)"("Item Symbols"=w295) -> ()  [unwired: 2 in, 2 out]
          }
          frame Default {
          }
        }
      }
      event "DB Camera Config": Value Change {
        # "Show or hide the cluster of controls, store in ini file"
        n202 = event-data() -> ("NewVal"=w300:bool)  [unwired: 1 in]
        n203 = case shown="False" w300 {
          tunnel: w299 -> [w309 _]
          tunnel: [w302 w320] -> w298
          tunnel: w297 -> [w301 w320]
          frame False {
            w316 = "Camera"
            w319 = FALSE ("Visible")
            n204 = local read "Camera Settings"() -> (w308:T2)
            n205 = Index Array(array=w309) -> (element=w312:cluster{string[]})  [unwired: 1 in]
            n206 = Unbundle(w308) -> ("Frame Rate"=w307:i32, "Compression"=w306:i32, "Size"=w310:u16)
            n207 = Unbundle(w312) -> (w311:string[])
            n208 = Index Array(array=w311, index=w310) -> (element=w305:string)
            n209 = call-poly <vilib>:"Write Key.vi"("section"=w316, "value"=w305, "key"="Size", "refnum"=w301) -> ("refnum out"=w318:T15)  [unwired: 2 in, 5 out]
            n210 = call-poly <vilib>:"Write Key.vi"("section"=w316, "value"=w307, "key"="FrameRate", "refnum"=w318) -> ("refnum out"=w317:T15)  [unwired: 1 in, 6 out]
            n211 = property on="Camera Settings" class="Clust (strict)"("Visible"=w319) -> ()  [unwired: 2 in, 2 out]
            n212 = local write "DB Camera Config"(w319) -> ()
            n213 = call-poly <vilib>:"Write Key.vi"("section"=w316, "value"=w306, "key"="Compression", "refnum"=w317) -> ("refnum out"=w303:T15)  [unwired: 1 in, 6 out]
            n214 = call <vilib>:"Close Config Data.vi"("refnum"=w303) -> ("file path"=w304:path)  [unwired: 2 in, 8 out]
            n215 = call <vilib>:"Open Config Data.vi"("configuration file path"=w304) -> ("refnum"=w302:T15)  [unwired: 8 in, 2 out]
          }
          frame True {
            n216 = property on="Camera Settings" class="Clust (strict)"("Visible"=TRUE) -> ()  [unwired: 2 in, 2 out]
          }
        }
      }
      event "Camera Settings": Value Change {
        # "Update summary string when any elements of DB camera change"
        n217 = event-data() -> ("NewVal"=w333:T2)  [unwired: 1 in]
        n218 = Index Array(array=w329) -> (element=w328:cluster{string[]})  [unwired: 1 in]
        n219 = Unbundle(w333) -> ("Frame Rate"=w324:i32, "Compression"=w323:i32, "Size"=w326:u16)
        n220 = Unbundle(w328) -> (w327:string[])
        n221 = Index Array(array=w327, index=w326) -> (element=w325:string)
        n222 = Format Into String(format string="%s   %dfps   %d%%", w325, w324, w323) -> (resulting string=w330:string)  [unwired: 2 in, 1 out]
        n223 = Build Array(w330) -> (w331:string[])
        n224 = property on="DB Camera Config" class="Bool (strict)"("Strings [4]"=w331) -> ()  [unwired: 2 in, 2 out]
      }
      event "Motor.Enable": Value Change {
        # "When the test mode otor enable helper is set, update that\ntree row item's value"
        n225 = event-data() -> ("NewVal"=w339:bool)  [unwired: 1 in]
        n226 = Unbundle("Motor") -> ("Value"=w338:dbl)  [unwired: 1 out]
        n227 = Select(t=w338, s=w339, f=0.0) -> (s? t:f=w336:dbl)
        n228 = call <vilib>:"NT Write Number.vi"("Numeric"=w336, "Name"=w335) -> ()  [unwired: 9 in, 1 out]
      }
      event "Test Slider": Value Change {
        # "When the test mode slider helper is set, update that\ntree row item's value"
        n229 = event-data() -> ("NewVal"=w342:dbl)  [unwired: 1 in]
        n230 = call <vilib>:"NT Write Number.vi"("Numeric"=w342, "Name"=w343) -> ()  [unwired: 9 in, 1 out]
      }
      event "On/Off": Value Change {
        # "When the test mode on/off helper value is set, update that\ntree row item's value"
        n231 = event-data() -> ("NewVal"=w347:bool)  [unwired: 1 in]
        n232 = Boolean To (0,1)(Boolean=w347) -> (0, 1=w346:i16)
        n233 = call <vilib>:"NT Write Number.vi"("Numeric"=w346, "Name"=w345) -> ()  [unwired: 9 in, 1 out]
      }
      event "Rev/Fwd": Value Change {
        # "When the test mode helper value for relays is set, update that\ntree row item's value"
        n234 = event-data() -> ("NewVal.Forward"=w355:bool, "NewVal.Reverse"=w354:bool)  [unwired: 1 in]
        n235 = Boolean To (0,1)(Boolean=w355) -> (0, 1=w351:i16)
        n236 = Boolean To (0,1)(Boolean=w354) -> (0, 1=w353:i16)
        n237 = Negate(x=w353) -> (-x=w352:i16)
        n238 = Add(x=w351, y=w352) -> (x+y=w350:i16)
        n239 = call <vilib>:"NT Write Number.vi"("Numeric"=w350, "Name"=w349) -> ()  [unwired: 9 in, 1 out]
      }
      event "Test Ring": Value Change {
        # "When a test mode helper value is selected from the ring,\nset the tree item's variable to the string value"
        n240 = event-data() -> ("NewVal"=w359:u16)  [unwired: 1 in]
        n241 = property on="Test Ring" class="Ring (strict)"() -> ("Strings []"=w360:string[])  [unwired: 2 in, 2 out]
        n242 = Index Array(array=w360, index=w359) -> (element=w358:string)
        n243 = call <vilib>:"NT Write String.vi"("String"=w358, "Name"=w357) -> ()  [unwired: 9 in, 1 out]
      }
      event "Rec Mode": Value Change {
        # "Update globals for recording mode and path to read log from.\nClear when logging and let NetworkTables set path for vision to\nuse."
        n244 = event-data() -> ("NewVal"=w370:enum32{"Stop", "Record", "Playback"})  [unwired: 1 in]
        n245 = global write "WPI_DashboardLogging Global.vi" "Logging Filename"(path "") -> ()
        n246 = case shown="\"Playback\"" w370 {
          tunnel: w369 -> [_ w372 w380]
          tunnel: [_ _ w379] -> w366
          tunnel: [_ _ w378] -> _
          tunnel: w364 -> [_ _ w376]
          tunnel: cluster{i32, i32} {-250, 170} -> [_ _ w375]
          tunnel: [_ _ T18 {"Image Size"=TRUE, "Image Type"=TRUE, "Pixel Value"=TRUE, "ROI Information"=TRUE, "Zoom Factor"=FALSE} ("Image Information Shown:All Elements")] -> w362
          tunnel: [_ _ TRUE ("Zoom Factor")] -> w361
          frame Default {
          }
          frame "Stop", "Record" {
            # "Place Window too"
            n247 = invoke class="VI" method="FP.Close"(reference=w372) -> (reference out=w371:refnum<vi>)  [unwired: 2 in, 2 out]
            n248 = invoke class="VI" method="Abort VI"(reference=w371) -> ()  [unwired: 2 in, 3 out]
          }
          frame "Playback" {
            n249 = call "Open Playback Panel.vi"("Offset"=w375, "DB VI Ref"=w376, "Playback in"=w380) -> ("Playback out"=w377:refnum<vi>)  [unwired: 8 in]
            n250 = register-events(w377) -> (reference out=w379:refnum<event-registration>, error out=w378:errorcluster)  [unwired: 2 in]
          }
        }
        n251 = global write "WPI_DashboardLogging Global.vi" "Recording"(w370) -> ()
        n252 = property on="Camera Image" class="ImageControl"("Image Information Shown"=w362, "Image Information Visible"=w361) -> ()  [unwired: 2 in, 2 out]
        n253 = call <vilib>:"WPI_DashboardNT Log FieldName Cache.vi"("Operation"=enum16{"Lookup/Add", "Index", "Clear"}."Clear") -> ()  [unwired: 8 in, 3 out]
      }
      event Panel Close {
        w381 = enum32{"Stop", "Record", "Playback"}."Stop" ("Rec Mode")
        # "Playback window has been closed, abort"
        n254 = event-data() -> ()  [unwired: 1 in, 4 out]
        n255 = local write "Rec Mode"(w381) -> ()
        n256 = global write "WPI_DashboardLogging Global.vi" "Recording"(w381) -> ()
      }
      event Panel Close {
        # "Abort playback window and ourself"
        n257 = event-data() -> ()  [unwired: 1 in, 4 out]
        n258 = invoke class="VI" method="FP.Close"(reference=w386) -> (reference out=w385:refnum<vi>)  [unwired: 2 in, 2 out]
        n259 = invoke class="VI" method="Abort VI"(reference=w385) -> (error out=w384:errorcluster)  [unwired: 2 in, 2 out]
        n260 = invoke class="VI" method="Abort VI"(error in=w384) -> ()  [unwired: 2 in, 3 out]
      }
      event "Vision": Value Change {
        # "Enable/Disable Compression slider.\nHW USB is hard-coded into the camera"
        n261 = event-data() -> ("NewVal"=w392:u16)  [unwired: 1 in]
        n262 = Equal?(x=w392, y=u32 2 ("milliseconds to wait")) -> (x = y?=w390:bool)
        n263 = Select(t=T19."Disabled and Grayed Out" ("Disabled"), s=w390, f=T19."Enabled" ("Disabled")) -> (s? t:f=w387:T19)
        n264 = property on="Compression" class="Slide (strict)"("DisabledEnum"=w387) -> ()  [unwired: 2 in, 2 out]
      }
    }
  }
  n265 = while {
    tunnel: w37 -> [w395]
    i -> [w398]
    stop <- FALSE stop-if-true
    n266 = Wait (ms)(milliseconds to wait=u32 100) -> ()  [unwired: 1 out]
    n267 = case shown="\"Playback\"" "Rec Mode" {
      tunnel: w398 -> [_ _ w413]
      tunnel: [u32 2829099 ("Base Color") u32 11141120 ("Target Color") w402] -> w394
      frame "Stop", Default {
        # "Reset the color, extra updates don't cost much"
      }
      frame "Record" {
      }
      frame "Playback" {
        # "Playback"
        n268 = Quotient & Remainder(x=w413, y=u32 50 ("milliseconds to wait")) -> (x-y*floor(x/y)=w409:u32)  [unwired: 1 out]
        n269 = Divide(x=w409, y=u32 50 ("milliseconds to wait")) -> (x/y=w406:dbl)
        n270 = Multiply(x=6.283185307179586, y=w406) -> (x*y=w411:dbl)
        n271 = Sine(x=w411) -> (sin(x)=w410:dbl)
        n272 = Absolute Value(x=w410) -> (abs(x)=w403:dbl)
        n273 = call "Interpolate RGB Color.vi"("Proportion"=w403, "Target Color"=u32 30976, "Base Color"=u32 2829099) -> ("Result Color"=w402:u32)  [unwired: 8 in]
      }
    }
    n274 = property class="Pane"(reference=w395, "PaneColor"=w394) -> ()  [unwired: 1 in, 2 out]
  }
  n275 = TCP Create Listener(10:u16 1741 ("timeout ms (25000)")) -> (3:w1:refnum<k5>)  [unwired: 4 in, 2 out]
  n276 = while {
    tunnel: w1 -> [w415]
    stop <- FALSE stop-if-true
    n277 = TCP Wait On Listener(11:w415) -> (4:w414:refnum<k5>)  [unwired: 3 in, 4 out]
    n278 = local write "TCP"(w414) -> ()
  }
  n279 = property on="On/Off" class="Bool (strict)"("Visible"=w6) -> ()  [unwired: 2 in, 2 out]
  n280 = property on="Motor" class="Clust (strict)"("Visible"=w6) -> ()  [unwired: 2 in, 2 out]
  n281 = property on="Progress" class="Clust (strict)"("Visible"=w6) -> ()  [unwired: 2 in, 2 out]
  n282 = property on="Test Ring" class="Ring (strict)"("Visible"=w6) -> ()  [unwired: 2 in, 2 out]
  n283 = property on="Rev/Fwd" class="Clust (strict)"("Visible"=w6) -> ()  [unwired: 2 in, 2 out]
  n284 = property on="Camera Settings" class="Clust (strict)"("Visible"=w6) -> ()  [unwired: 2 in, 2 out]
  n285 = local write "DB Camera Config"(w6) -> ()
  n286 = global write "WPI_DashboardLogging Global.vi" "Recording"(w31) -> ()
  n287 = local write "Rec Mode"(w31) -> ()
